vi "EndOfPathHandler.vi"(4 "DistanceToEnd":dbl, 6 "CurrentVel":dbl, 8 "MaxAccel":dbl, 9 "MaxVel":dbl, 10 "RobotLocation":cluster{dbl, dbl}, 11 "Path":cluster{"x":dbl, "y":dbl}[](array[cluster])=[{"x"=0.0, "y"=10.0}, {"x"=0.0, "y"=80.0}, {"x"=85.0, "y"=140.0}, {"x"=85.0, "y"=20.0}, {"x"=40.0, "y"=15.0}]) -> (0 "Done":bool, 1 "Override":bool, 2 "ExtraPowerOut":dbl, 3 "VelOut":dbl)   [LabVIEW 2017]
doc: "The end of path handler says when the robot is done traveling the path. It also outputs the velocity the robot should travel at.\n\"But wait!\" you say, \"I thought that was what the MaxVel control was for\". Yes, but the end of path handler outputs 0 vel when the robot gets to the\ndistance it should start deaccelerating (at the END of the PATH). (this vel gets fed into a rate limiter so it obeys max acceleration). This is how it deaccelerates. \n It also outputs a boolean named Override, which tells the robot to stop using a PIDF controller and travel at a constant, slow, speed. This is to try and prevent\nOvershoot at the end. That is a bad solution."
panel:
  in  "PID gains":T1 {"derivative time (Td, min)" format="%.3f"; "integral time (Ti, min)" format="%.3f"; "proportional gain (Kc)" format="%.3f"}
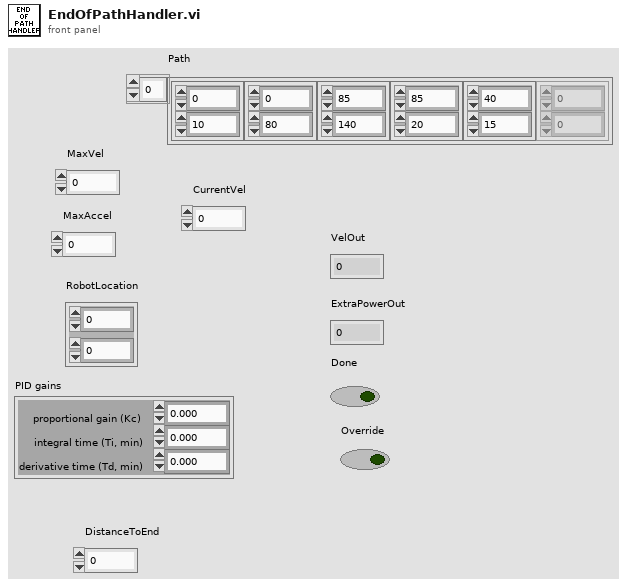
[diagram p1: front panel]
types:
  T1 = cluster{"proportional gain (Kc)":dbl, "integral time (Ti, min)":dbl, "derivative time (Td, min)":dbl}
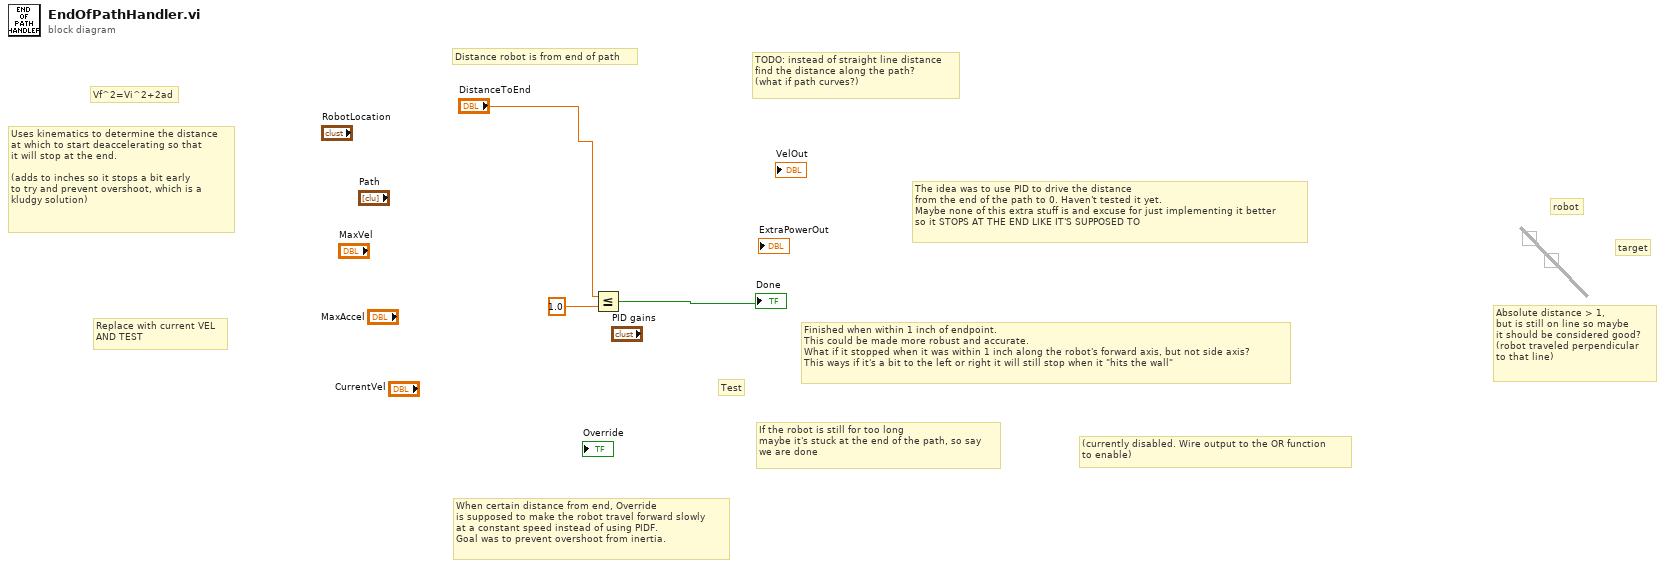
[diagram p0: block diagram]
diagram:
  # "Absolute distance > 1,\nbut is still on line so maybe\nit should be considered good?\n(robot traveled perpendicular\nto that line)"
  # "robot"
  # "target"
  # "Finished when within 1 inch of endpoint.\nThis could be made more robust and accurate.\nWhat if it stopped when it was within 1 inch along the robot's forward axis, but not side axis?\nThis ways if it's a bit to the left or right it will still stop when it \"hits the wall\""
  # "When certain distance from end, Override\nis supposed to make the robot travel forward slowly\nat a constant speed instead of using PIDF.\nGoal was to prevent overshoot from inertia."
  # "(currently disabled. Wire output to the OR function\nto enable)"
  # "If the robot is still for too long\nmaybe it's stuck at the end of the path, so say\nwe are done"
  # "The idea was to use PID to drive the distance\nfrom the end of the path to 0. Haven't tested it yet.\nMaybe none of this extra stuff is and excuse for just implementing it better\nso it STOPS AT THE END LIKE IT'S SUPPOSED TO"
  # "TODO: instead of straight line distance\nfind the distance along the path?\n(what if path curves?)"
  # "Uses kinematics to determine the distance\nat which to start deaccelerating so that\nit will stop at the end.\n\n(adds to inches so it stops a bit early\nto try and prevent overshoot, which is a\nkludgy solution)"
  # "Distance robot is from end of path"
  # "Test"
  # "Replace with current VEL\nAND TEST"
  # "Vf^2=Vi^2+2ad"
  n1 = Less Or Equal?(x="DistanceToEnd", y=1.0) -> (x <= y?=→"Done":bool)
